vi "NotificationGetFleetSitesRequest_Create.vi"(7 "Header":T1, 8 "error in (no error)":errorcluster, 11 "ReplyTo":string) -> (0 "error out":errorcluster, 3 "Message":T3)   [LabVIEW 2017]
uses:
  <vilib>/addons/InsightCM/MessageBus/Base/controls/Message.ctl
  <vilib>/addons/InsightCM/MessageBus/Base/controls/MessageHeader.ctl
  <vilib>/addons/InsightCM/MessageBus/Base/controls/KeyValuePair.ctl
  <vilib>/addons/InsightCM/MessageBus/Base/controls/MessageClassType.ctl
  <vilib>/addons/InsightCM/Utilities/PropertyHelpers/PropertyHelpers.lvlib
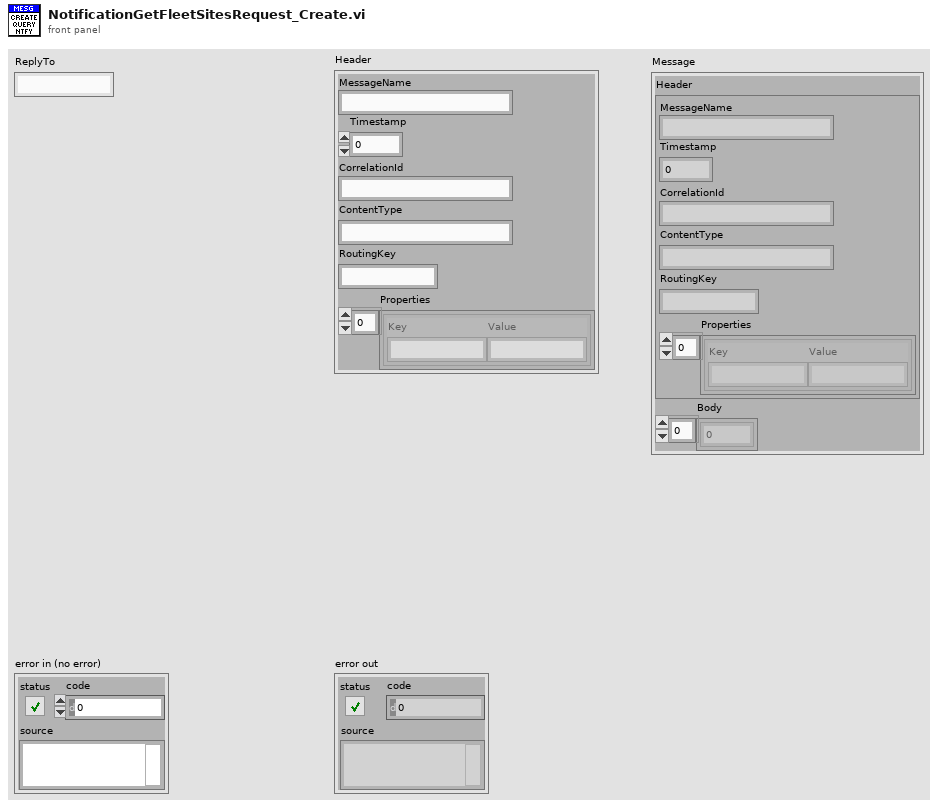
[diagram p1: front panel]
types:
  T1 = typedef "MessageHeader.ctl" = cluster{"MessageName":string, "Timestamp":i64, "CorrelationId":string, "ContentType":string, "RoutingKey":string, "Properties":T2[]}
  T2 = typedef "KeyValuePair.ctl" = cluster{"Key":string, "Value":string}
  T3 = typedef "Message.ctl" = cluster{"Header":T1, "Body":u8[]}
  T4 = typedef "MessageClassType.ctl" = enum16{"Request", "Response", "Broadcast", "RoutedMessage"}
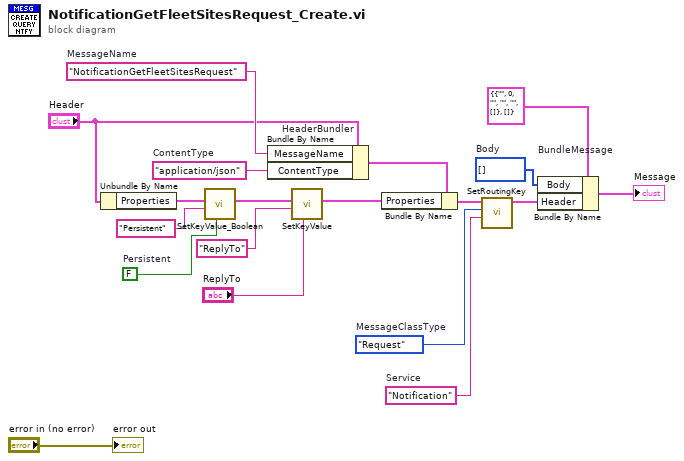
[diagram p0: block diagram]
diagram:
  w18 = u8[] []  # Body
  w16 = MessageClassType."Request"  # MessageClassType
  w1 = "Notification"  # Service
  w11 = FALSE  # Persistent
  w17 = "NotificationGetFleetSitesRequest"  # MessageName
  w14 = "application/json"  # ContentType
  n1 = Unbundle By Name("Header") -> ("Properties"=w13:T2[])
  n2 = call <vilib>:"SetKeyValue_Boolean.vi"("value"=w11, "key"="Persistent" ("Key"), "key value pairs"=w13) -> ("key value pairs out"=w9:T2[])  [unwired: 8 in]
  n3 = Bundle By Name "HeaderBundler"(cluster="Header", "MessageName"=w17, "ContentType"=w14) -> (w7:T1)
  n4 = call <vilib>:"SetKeyValue.vi"("value"="ReplyTo", "key"="ReplyTo" ("Key"), "key value pairs"=w9) -> ("key value pairs out"=w6:T2[])  [unwired: 8 in]
  n5 = Bundle By Name(cluster=w7, "Properties"=w6) -> (w8:T1)
  n6 = call <vilib>:"SetRoutingKey.vi"("SendTo"=w1, "MessageClassType"=w16, "Message Header in"=w8) -> ("Message Header out"=w10:T1)  [unwired: 8 in]
  n7 = Bundle By Name "BundleMessage"(cluster=T3 {"Header"={"MessageName"="", "Timestamp"=0, "CorrelationId"="", "ContentType"="", "RoutingKey"="", "Properties"=[]}, "Body"=[]} ("Message"), "Body"=w18, "Header"=w10) -> (→"Message":T3)
  "error out" <- "error in (no error)"
